vi "Set RTB Selection Text Alignmentvi.vi"(8 "Error In":errorcluster, 9 "Text Alignment":i32(ring) items=["Left", "Right", "Center"], 11 ".NET RTB Refnum in":refnum<k24>) -> (0 "Error Out":errorcluster, 3 ".NET RTB Refnum out":refnum<k24>)   [LabVIEW 2021, in "Rich Text Box.lvlib"]
uses:
  Rich Text Box.lvlib
  System.Windows.Forms
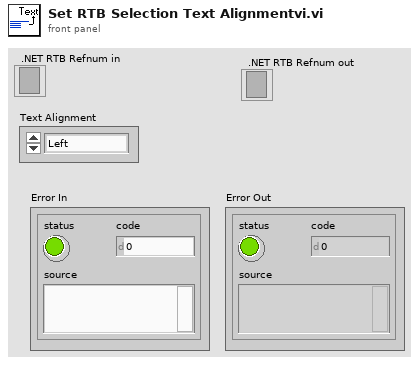
[diagram p1: front panel]
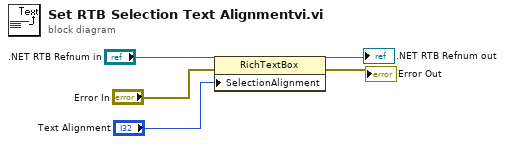
[diagram p0: block diagram]
diagram:
  n1 = property class="RichTextBox"(reference=".NET RTB Refnum in", error in="Error In", "SelectionAlignment"="Text Alignment") -> (reference out=→".NET RTB Refnum out":refnum<k24>, error out=→"Error Out":errorcluster)
